vi "Temp to API Value.vi"(10 "Color Temp":dbl) -> (2 "API Temp":dbl)   [LabVIEW 2022 SP3, in "TouchControl.lvlib" / "LightsPanel.lvclass"]
uses:
  LightsPanel.lvclass
  <vilib>/Analysis/NI_AALPro.lvlib
panel:
  out "offset":dbl
  out "power":dbl
  out "amplitude":dbl
  out "Best Power Fit":dbl[](array[numeric])
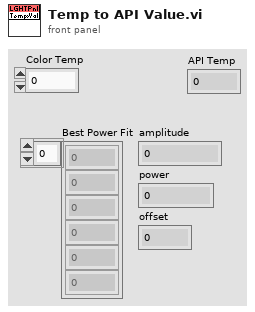
[diagram p1: front panel]
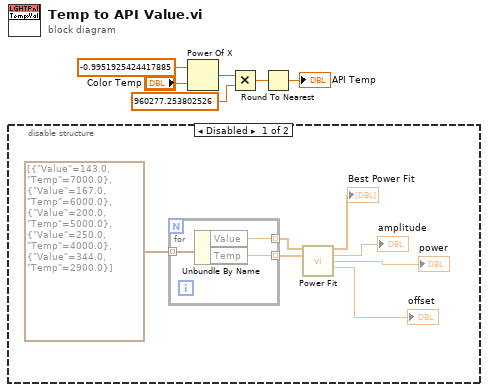
[diagram p0: block diagram]
diagram:
  n1 = disable-structure shown="Disabled" {
    frame Disabled {
      n2 = for {
        tunnel: cluster{"Value":dbl, "Temp":dbl}[] [{"Value"=143.0, "Temp"=7000.0}, {"Value"=167.0, "Temp"=6000.0}, {"Value"=200.0, "Temp"=5000.0}, {"Value"=250.0, "Temp"=4000.0}, {"Value"=344.0, "Temp"=2900.0}] -> [w16] mode=indexing
        tunnel: [w15] -> w12 mode=indexing
        tunnel: [w14] -> w11 mode=indexing
        n3 = Unbundle By Name(w16) -> ("Value"=w15:dbl, "Temp"=w14:dbl)
      }
      n4 = call <vilib>:"Power Fit.vi"("Y"=w12, "X"=w11) -> ("Best Power Fit"=→"Best Power Fit":dbl[], "amplitude"=→"amplitude":dbl, "power"=→"power":dbl, "offset"=→"offset":dbl)  [unwired: 8 in, 2 out]
    }
    frame Enabled {
    }
  }
  n5 = Power Of X(1:"Color Temp", 2:-0.9951925424417885 ("power")) -> (0:w6:dbl)
  n6 = Multiply(x=w6, y=960277.253802526 ("amplitude")) -> (x*y=w4:dbl)
  n7 = Round To Nearest(number=w4) -> (nearest integer value=→"API Temp":dbl)
